vi "Convert Bool Array to Cluster BLOB.vi"(8 "error in (no error)":errorcluster, 10 "Cluster Bool Array out":bool[](array[boolean])) -> (0 "error out":errorcluster, 2 "Cluster BLOB":u8[](array[numeric]))   [LabVIEW 2018, in "Scalar IO Operations.lvlib"]
uses:
  Scalar IO Operations.lvlib
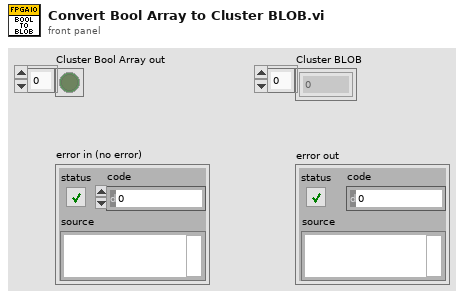
[diagram p1: front panel]
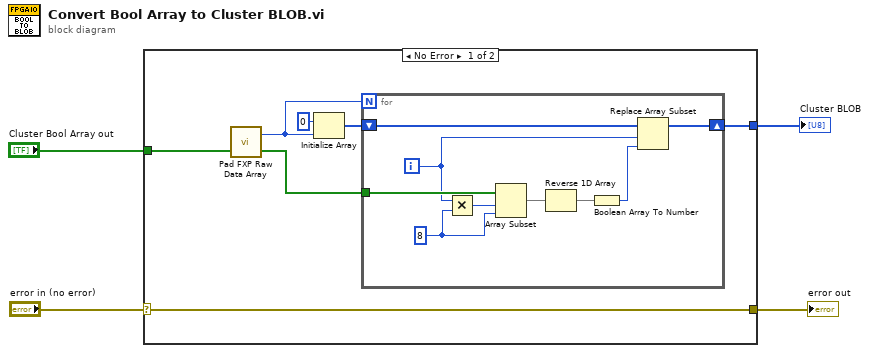
[diagram p0: block diagram]
diagram:
  n1 = case shown="No Error" "error in (no error)" {
    selector: "error in (no error)" -> [w11 w21]
    tunnel: [w11 w21] -> w3
    tunnel: "Cluster Bool Array out" -> [w7 _]
    tunnel: [w8 _] -> w1
    frame No Error {
      n2 = call "Pad FXP Raw Data Array.vi"("Cluster Bool Array in"=w7) -> ("Cluster Bool Array out"=w6:bool[], "Size (bytes)"=w5:i32)  [unwired: 1 in]
      n3 = Initialize Array(u8 0, w5) -> (w9:u8[])
      n4 = for {
        N: w5 -> [_]
        tunnel: w6 -> [w20]
        shift-right: [w16] -> w8
        shift-left: w9 -> [w17]
        i -> [w13]
        w12 = 8 ("length")
        n5 = Multiply(x=w13, y=w12) -> (x*y=w15:i32)
        n6 = Array Subset(array=w20, index=w15, length=w12) -> (w19:bool[])
        n7 = Reverse 1D Array(array=w19) -> (reversed array=w18:bool[])
        n8 = Boolean Array To Number(Boolean array=w18) -> (number=w14:u8)
        n9 = Replace Array Subset(array=w17, new element=w14, index=w13) -> (w16:u8[])
      }
    }
    frame Error {
    }
  }
  "error out" <- w3
  "Cluster BLOB" <- w1
